vi "GEM_BANK_ARRAY_Add_Data.vi"(8 "error in (no error)":errorcluster, 10 "GEM BANK Cluster":T1, 11 "LVBANKARRAY in":refnum<class "GEM_BANK_ARRAY.lvclass">) -> (0 "error out":errorcluster, 3 "LVBANKARRAY out":refnum<class "GEM_BANK_ARRAY.lvclass">)   [LabVIEW 2018, in "GEM_BANK_ARRAY.lvclass"]
uses:
  GEM_BANK_ARRAY.lvclass
  GEM_BANK_CLUSTER_typedef.ctl
  GEM_DATA_cluster_typedef.ctl
  GEM_BANK_ARRAY.lvclass/GEM_BANK_ARRAY.ctl
  GEM_BANK.lvclass
  GEM_BANK.lvclass/GEM_BANK.ctl
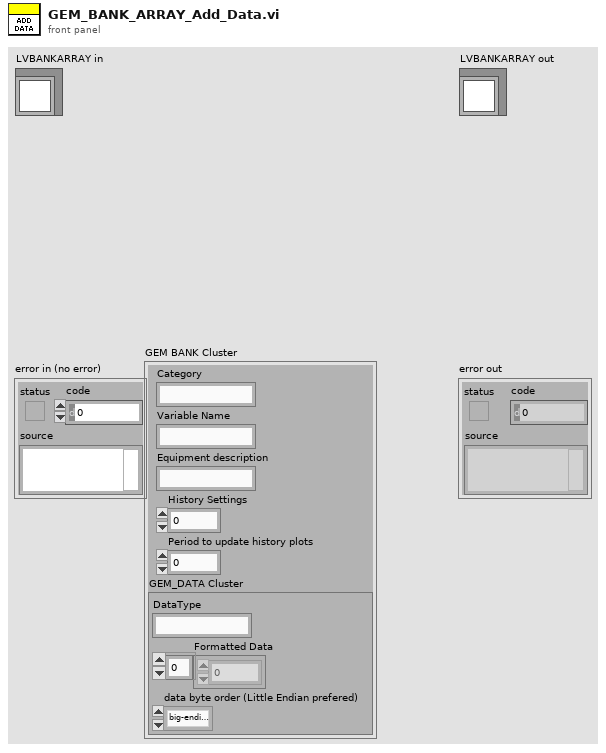
[diagram p1: front panel]
types:
  T1 = typedef "GEM_BANK_CLUSTER_typedef.ctl" = cluster{"Category":string, "Variable Name":string, "Equipment description":string, "History Settings":u16, "Period to update history plots":u16, "GEM_DATA Cluster":T2}
  T2 = typedef "GEM_DATA_cluster_typedef.ctl" = cluster{"DataType":string, "Formatted Data":u8[], "data byte order (Little Endian prefered)":enum16{"big-endian, network order", "native, host order", "little-endian"}}
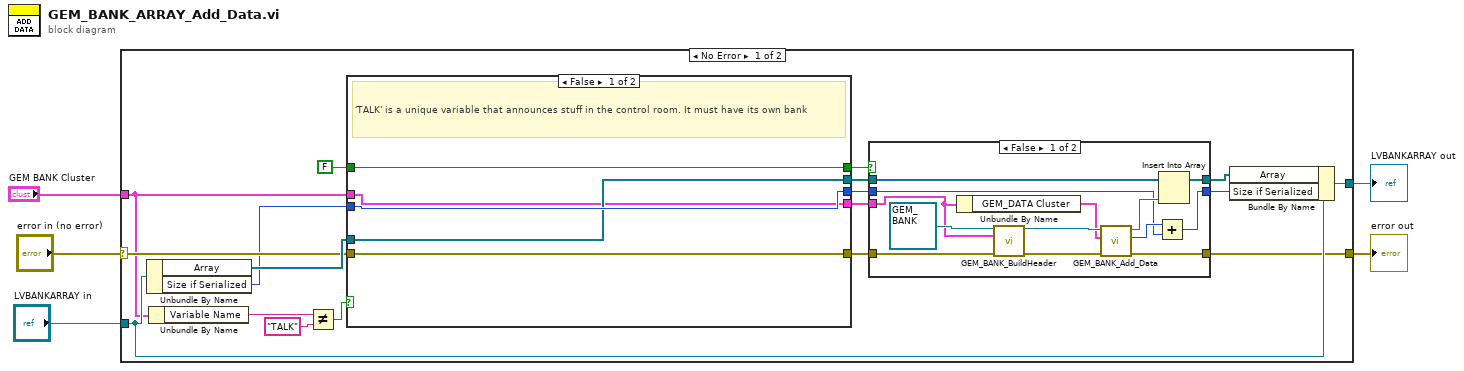
[diagram p0: block diagram]
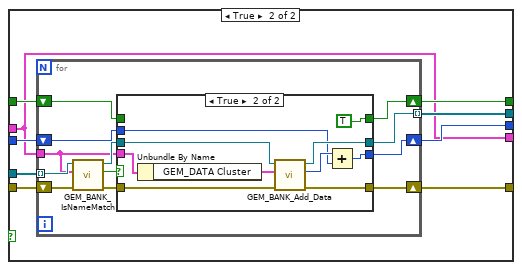
[diagram p2: hidden frame]
diagram:
  n1 = case shown="No Error" "error in (no error)" {
    selector: "error in (no error)" -> [w22 w80]
    tunnel: [w14 w80] -> w1
    tunnel: "LVBANKARRAY in" -> [w20 w81]
    tunnel: [w21 w81] -> w3
    tunnel: "GEM BANK Cluster" -> [w7 _]
    frame No Error {
      n2 = Unbundle By Name(w20) -> ("Array"=w23:refnum<class "GEM_BANK.lvclass">[], "Size if Serialized"=w13:u32)
      n3 = Unbundle By Name(w7) -> ("Variable Name"=w10:string)
      n4 = Not Equal?(x=w10, y="TALK") -> (x != y?=w8:bool)
      n5 = case shown="False" w8 {
        tunnel: w23 -> [w26 w37]
        tunnel: w22 -> [w24 w36]
        tunnel: FALSE -> [w28 w35]
        tunnel: [w28 w34] -> w18
        tunnel: [w26 w33] -> w17
        tunnel: [w24 w32] -> w15
        tunnel: w13 -> [w27 w31]
        tunnel: [w27 w30] -> w12
        tunnel: w7 -> [w25 w29]
        tunnel: [w25 w29] -> w6
        frame False {
          # "'TALK' is a unique variable that announces stuff in the control room. It must have its own bank"
        }
        frame True {
          n6 = for {
            tunnel: w37 -> [w49] mode=indexing
            tunnel: [w45] -> w33 mode=indexing
            shift-right: [w43] -> w32
            shift-left: w36 -> [w48]
            shift-right: [w41] -> w34
            shift-left: w35 -> [w42]
            tunnel: w29 -> [w40]
            shift-right: [w38] -> w30
            shift-left: w31 -> [w39]
            n7 = call "GEM_BANK_IsNameMatch.vi"("error in (no error)"=w48, "GEM_BANK Cluster"=w40, "LVBANK in"=w49) -> ("error out"=w44:errorcluster, "BANK MATCHES"=w47:bool, "LVBANK out"=w46:refnum<class "GEM_BANK.lvclass">)  [unwired: 6 in]
            n8 = case shown="True" w47 {
              tunnel: w46 -> [w53 w63]
              tunnel: [w53 w62] -> w45
              tunnel: w44 -> [w52 w61]
              tunnel: [w52 w60] -> w43
              tunnel: w42 -> [w51 _]
              tunnel: [w51 TRUE] -> w41
              tunnel: w40 -> [_ w58]
              tunnel: w39 -> [w50 w55]
              tunnel: [w50 w54] -> w38
              frame False {
              }
              frame True {
                n9 = Unbundle By Name(w58) -> ("GEM_DATA Cluster"=w57:T2)
                n10 = call "GEM_BANK_Add_Data.vi"("error in (no error)"=w61, "GEM_DATA"=w57, "LVBANK in"=w63) -> ("error out"=w60:errorcluster, "Bank Size (bytes)"=w56:u32, "LVBANK out"=w62:refnum<class "GEM_BANK.lvclass">)  [unwired: 6 in]
                n11 = Add(x=w56, y=w55) -> (x+y=w54:u32)
              }
            }
          }
        }
      }
      n12 = case shown="False" w18 {
        tunnel: w17 -> [w76 w79]
        tunnel: [w75 w79] -> w16
        tunnel: w15 -> [w73 w78]
        tunnel: [w70 w78] -> w14
        tunnel: w6 -> [w68 _]
        tunnel: w12 -> [w64 w77]
        tunnel: [w65 w77] -> w11
        frame False {
          n13 = Unbundle By Name(w68) -> ("GEM_DATA Cluster"=w67:T2)
          n14 = call "GEM_BANK_BuildHeader.vi"("LVBANK in"=refnum<class "GEM_BANK.lvclass"> refnum, "GEM BANK cluster"=w68, "error in (no error)"=w73) -> ("LVBANK out"=w72:refnum<class "GEM_BANK.lvclass">, "error out"=w71:errorcluster)  [unwired: 11 in]
          n15 = call "GEM_BANK_Add_Data.vi"("error in (no error)"=w71, "GEM_DATA"=w67, "LVBANK in"=w72) -> ("error out"=w70:errorcluster, "Bank Size (bytes)"=w66:u32, "LVBANK out"=w69:refnum<class "GEM_BANK.lvclass">)  [unwired: 6 in]
          n16 = Add(x=w66, y=w64) -> (x+y=w65:u32)
          n17 = Insert Into Array(array=w76, new element=w69) -> (w75:refnum<class "GEM_BANK.lvclass">[])  [unwired: 1 in]
        }
        frame True {
        }
      }
      n18 = Bundle By Name(cluster=w20, "Array"=w16, "Size if Serialized"=w11) -> (w21:refnum<class "GEM_BANK_ARRAY.lvclass">)
    }
    frame Error {
    }
  }
  "error out" <- w1
  "LVBANKARRAY out" <- w3
